vi "Keep or Discard.vi"(10 "match?":bool, 11 "filter":refnum<class "Filter.lvclass">) -> (2 "discard?":bool, 3 "dup filter":refnum<class "Filter.lvclass">)   [LabVIEW 2018, in "GLog.lvlib" / "Filter.lvclass"]
uses:
  Filter.lvclass
  Filter.lvclass/Filter.ctl
panel:
  # "Connector Pane"
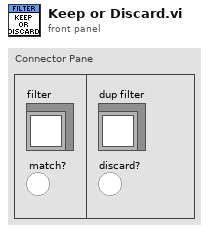
[diagram p1: front panel]
types:
  T1 = typedef "GLog.lvlib/Match Behavior.ctl" = enum16{"Keep", "Discard"}
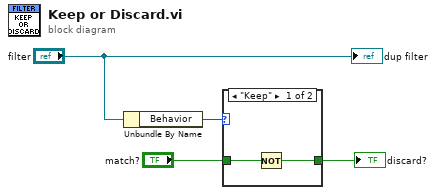
[diagram p0: block diagram]
diagram:
  n1 = Unbundle By Name("filter") -> ("Behavior"=w1:T1)
  n2 = case shown="\"Keep\"" w1 {
    tunnel: [w5 w7] -> w3
    tunnel: "match?" -> [w6 w7]
    frame "Keep" {
      n3 = Not(x=w6) -> (.not. x?=w5:bool)
    }
    frame "Discard" {
    }
  }
  "discard?" <- w3
  "dup filter" <- "filter"
